vi "Read Double Float 1D Value.vi"(8 "error in (no error)":errorcluster, 11 "Abs_Extend1D Float in":refnum<class "Abs_Extended Float 1D.lvclass">) -> (0 "error out":errorcluster, 2 "Double1D":dbl[](array[numeric]), 3 "Abs_Extend1D Float out":refnum<class "Abs_Extended Float 1D.lvclass">)   [LabVIEW 2021, in "Abs_Extended Float 1D.lvclass"]
uses:
  Abs_Extended Float 1D.lvclass
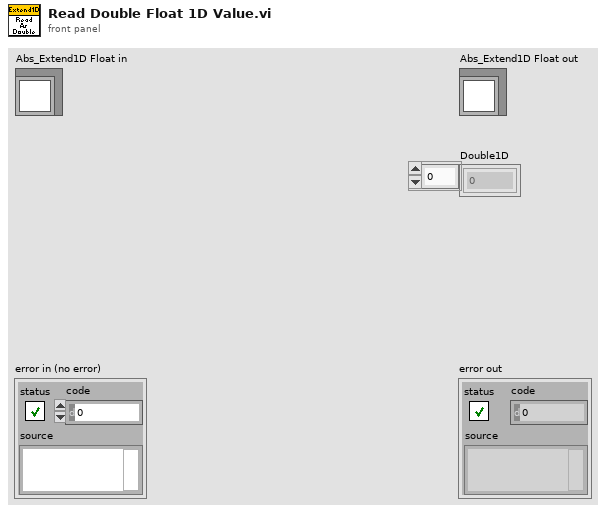
[diagram p1: front panel]
types:
  T1 = typedef "Abs_Extended Float 1D.lvclass/Type.ctl" = ext[]
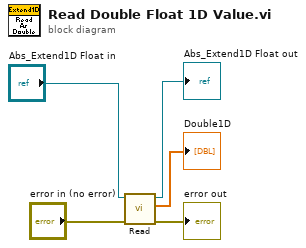
[diagram p0: block diagram]
diagram:
  n1 = call-dynamic "Read.vi"("error in (no error)"="error in (no error)", "Double Float.lvclass_340760 in"="Abs_Extend1D Float in") -> ("error out"=→"error out":errorcluster, "Value"=→"Double1D":T1, "Double Float.lvclass_340760 out"=→"Abs_Extend1D Float out":refnum<class "Abs_Extended Float 1D.lvclass">)  [unwired: 7 in]
